vi "is abstract node.vi"(8 "error in":errorcluster, 11 "Engine Parent Editor Node in":refnum<class "Engine Parent Editor Node.lvclass">) -> (0 "error out":errorcluster, 2 "abstract":bool, 3 "Engine Parent Editor Node out":refnum<class "Engine Parent Editor Node.lvclass">)   [LabVIEW 2013, in "PL Framework Configuration Tool.lvlib" / "Engine Parent Editor Node.lvclass"]
uses:
  Engine Parent Editor Node.lvclass
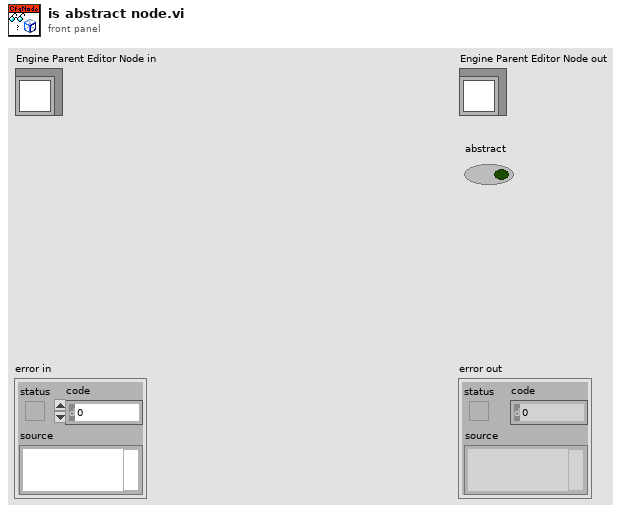
[diagram p1: front panel]
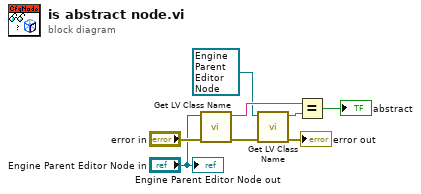
[diagram p0: block diagram]
diagram:
  n1 = call <vilib>:"Get LV Class Name.vi"("error in (no error)"="error in", "object"="Engine Parent Editor Node in") -> ("error out"=w4:errorcluster, "class name"=w6:string)  [unwired: 8 in]
  n2 = call <vilib>:"Get LV Class Name.vi"("error in (no error)"=w4, "object"=refnum<class "Engine Parent Editor Node.lvclass"> refnum ("Engine Parent Editor Node in")) -> ("error out"=→"error out":errorcluster, "class name"=w7:string)  [unwired: 8 in]
  n3 = Equal?(x=w6, y=w7) -> (x = y?=→"abstract":bool)
  "Engine Parent Editor Node out" <- "Engine Parent Editor Node in"
